vi "Test_Send_and_receive.vi"() -> ()   [LabVIEW 2020]
uses:
  <vilib>/Instr/_visa.llb/VISA Configure Serial Port (Serial Instr).vi
panel:
  in  "Send":bool
  in  "stop":bool
  in  "Target":u16
  in  "Cmd":T1(ring)=enum."Change Speed"
  out "read buffer":string
  out "hex string":string
  out "Full Cmd":string
  out "Error Code out":i32 format="%0.0f"
  in  "Serial Port 2":refnum<visa-resource-name>="COM8" caption="Serial Port"
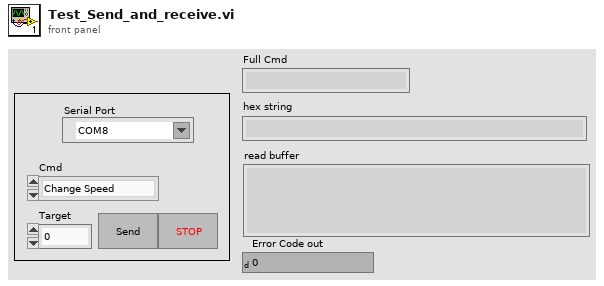
[diagram p1: front panel]
types:
  T1 = enum16{"Get Parameters", "Change Speed", "Change Inc"}
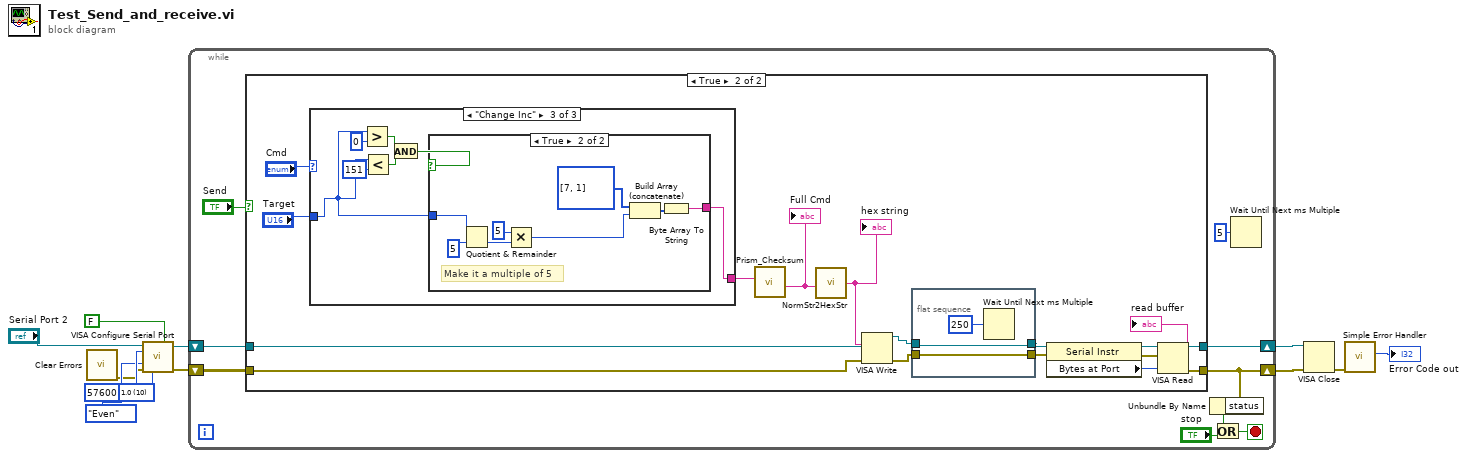
[diagram p0: block diagram]
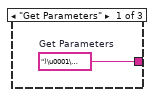
[diagram p3: hidden frame]
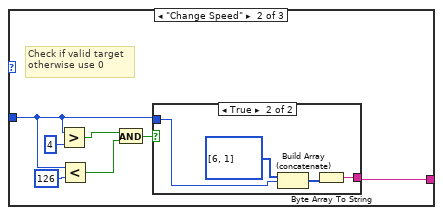
[diagram p4: hidden frame]
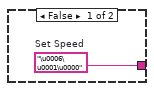
[diagram p5: hidden frame]
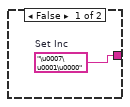
[diagram p6: hidden frame]
diagram:
  w9 = u16 10 items=["1.0"=10, "1.5"=15, "2.0"=20] ("stop bits (10: 1 bit)")
  n1 = call <vilib>:"Clear Errors.vi"() -> ("error out"=w1:errorcluster)  [unwired: 6 in, 1 out]
  n2 = call-poly "VISA Configure Serial Port"("VISA resource name"="Serial Port 2", "Enable Termination\nChar (T)"=FALSE ("Enable Termination\nChar (T)"), "baud rate (9600)"=u32 57600, "parity (0:none)"=enum16{"None", "Odd", "Even", "Mark", "Space"}."Even", "error in (no error)"=w1, "stop bits (10: 1 bit)"=w9) -> ("VISA resource name out"=w7:refnum<visa-resource-name>, "error out"=w6:errorcluster)  [unwired: 8 in]
  n3 = while {
    shift-right: [w19] -> w3
    shift-left: w7 -> [w21]
    shift-right: [w15] -> w2
    shift-left: w6 -> [w20]
    stop <- w17 stop-if-true
    n4 = case shown="True" "Send" {
      tunnel: w21 -> [w23 w40]
      tunnel: w20 -> [w22 w39]
      tunnel: [w23 w29] -> w19
      tunnel: [w22 w28] -> w15
      frame False {
      }
      frame True {
        n5 = case shown="\"Change Inc\"" "Cmd" {
          tunnel: "Target" -> [_ w46 w58]
          tunnel: [w41 w42 w57] -> w24
          frame "Get Parameters" {
            w41 = ")\u0001\u0000"  # Get Parameters
          }
          frame "Change Speed" {
            # "Check if valid target\notherwise use 0"
            n6 = Greater?(x=w46, y=u16 4) -> (0:w43:bool)
            n7 = Less?(x=w46, y=u16 126) -> (x < y?=w44:bool)
            n8 = And(x=w43, y=w44) -> (x .and. y?=w47:bool)
            n9 = case shown="True" w47 {
              tunnel: w46 -> [_ w53]
              tunnel: [w49 w50] -> w42
              frame False {
                w49 = "\u0006\u0001\u0000"  # Set Speed
              }
              frame True {
                n10 = Build Array (concatenate)(u8[] [6, 1] ("unsigned byte array"), w53) -> (w51:u16[])
                n11 = Byte Array To String(unsigned byte array=w51) -> (string=w50:string)
              }
            }
          }
          frame "Change Inc" {
            n12 = Greater?(x=w58, y=u16 0) -> (0:w55:bool)
            n13 = Less?(x=w58, y=u16 151) -> (x < y?=w56:bool)
            n14 = And(x=w55, y=w56) -> (x .and. y?=w54:bool)
            n15 = case shown="True" w54 {
              tunnel: w58 -> [_ w68]
              tunnel: [w61 w66] -> w57
              frame False {
                w61 = "\u0007\u0001\u0000"  # Set Inc
              }
              frame True {
                # "Make it a multiple of 5"
                n16 = Quotient & Remainder(x=w68, y=u16 5) -> (floor(x/y)=w65:u16)  [unwired: 1 out]
                n17 = Multiply(x=u16 5 ("y"), y=w65) -> (x*y=w63:u16)
                n18 = Build Array (concatenate)(u8[] [7, 1] ("unsigned byte array"), w63) -> (w62:u16[])
                n19 = Byte Array To String(unsigned byte array=w62) -> (string=w66:string)
              }
            }
          }
        }
        n20 = call "Prism_Checksum.vi"("ID +DB+ Data"=w24) -> ("Full Cmd"=w38:string)  [unwired: 10 in]
        "Full Cmd" <- w38
        n21 = call "NormStr2HexStr.vi"("string"=w38) -> ("hex string"=w37:string)
        "hex string" <- w37
        n22 = VISA Write(VISA resource name=w40, write buffer=w37, error in (no error)=w39) -> (VISA resource name out=w31:refnum<visa-resource-name>, error out=w30:errorcluster)  [unwired: 1 out]
        n23 = flat-sequence {
          tunnel: w31 -> [w71]
          tunnel: [w71] -> w27
          tunnel: w30 -> [w70]
          tunnel: [w70] -> w33
          frame #0 {
            n24 = Wait Until Next ms Multiple(millisecond multiple=u32 250) -> ()  [unwired: 1 out]
          }
        }
        n25 = property class="Serial Instr"(reference=w27, error in=w33) -> (reference out=w35:refnum<visa-resource-name>, error out=w36:errorcluster, "Bytes at Port"=w34:u32)
        n26 = VISA Read(VISA resource name=w35, byte count=w34, error in (no error)=w36) -> (VISA resource name out=w29:refnum<visa-resource-name>, read buffer=→"read buffer":string, error out=w28:errorcluster)  [unwired: 1 out]
      }
    }
    n27 = Unbundle By Name(w15) -> ("status"=w14:bool)
    n28 = Or(x=w14, y="stop") -> (x .or. y?=w17:bool)
    n29 = Wait Until Next ms Multiple(millisecond multiple=u32 5) -> ()  [unwired: 1 out]
  }
  n30 = VISA Close(VISA resource name=w3, error in (no error)=w2) -> (error out=w12:errorcluster)
  n31 = call <vilib>:"Simple Error Handler.vi"("error in (no error)"=w12) -> ("code out"=→"Error Code out":i32)  [unwired: 4 in, 4 out]
